vi "Begin.vi"() -> (0 "Error Out":errorcluster)   [LabVIEW 2014]
doc: "Called before other user functions, this VI is expected to open initial I/O refnums, load in file data, and do all program initialization. Notice that the <B>error out</B> terminal is simply used for data flow. Wiring it to other structures or subVIs ensures that this VI runs first."
uses:
  <vilib>/Rock Robotics/WPI/Joystick/WPI_JoystickDeviceEnum.ctl
  <vilib>/Rock Robotics/SystemInterfaces/DIO/FPGA_DIOChannel.ctl
  <vilib>/Rock Robotics/WPI/Solenoid/WPI_SolenoidChannel.ctl
  <vilib>/Rock Robotics/SystemInterfaces/Typedef/FPGA_TypedefDigitalModule.ctl
  <vilib>/Rock Robotics/WPI/Encoder/WPI_EncoderType.ctl
  <vilib>/Rock Robotics/SystemInterfaces/DIO/FPGA_DIOPWMChannel.ctl
  <vilib>/Rock Robotics/SystemInterfaces/AI/FPGA_AIGyroChannel.ctl
  <vilib>/Rock Robotics/SystemInterfaces/Typedef/FPGA_TypedefAnalogModuleForGyro.ctl
  <vilib>/Rock Robotics/SystemInterfaces/Typedef/FPGA_TypedefAnalogModule.ctl
  <vilib>/Rock Robotics/SystemInterfaces/AI/FPGA_AIChannel.ctl
  <vilib>/Rock Robotics/WPI/Solenoid/WPI_SolenoidValue.ctl
  <vilib>/Rock Robotics/WPI/CAN/TalonSRX/WPI_CANTalonSRX_APIControlMode.ctl
  <vilib>/Rock Robotics/WPI/Compressor/WPI_CompressorGetSetRefNum.vi
  <vilib>/Rock Robotics/WPI/Solenoid/WPI_SolenoidOpenDouble.vi
  <vilib>/Rock Robotics/WPI/Counter/WPI_CounterDigitalInputToDigitalSource.vi
  <vilib>/Rock Robotics/WPI/MotorControl/WPI_MotorControlOpen Talon.vi
  <vilib>/Rock Robotics/WPI/MotorControl/WPI_MotorControlOpenCANTalonSRX.vi
  <vilib>/Rock Robotics/WPI/RobotDrive/WPI_RobotDriveOpen4MotorWithExistingMotors.vi
  <vilib>/Rock Robotics/WPI/Solenoid/WPI_SolenoidSetEnum.vi
  <vilib>/Rock Robotics/WPI/RobotDrive/WPI_RobotDriveOpen4MotorWithCANTalonSRX.vi
  <vilib>/Rock Robotics/WPI/CAN/TalonSRX/WPI_CANTalonSRX_BrakeOverride.ctl
panel:
  # "Begin"
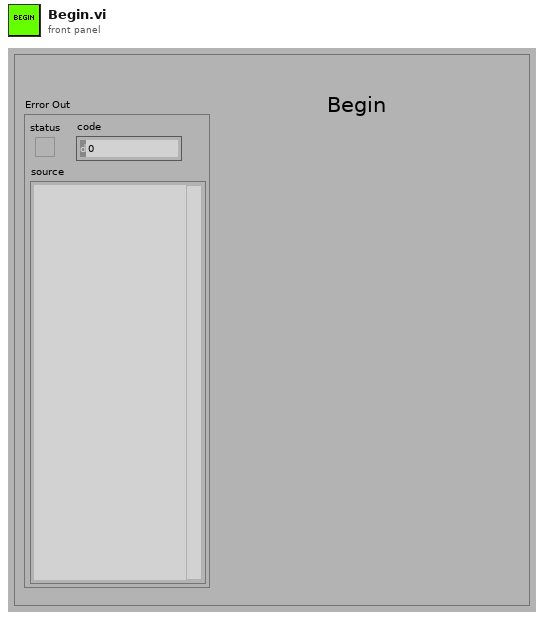
[diagram p1: front panel]
types:
  T1 = typedef "WPI_CANTalonSRX_APIControlMode.ctl" = enum8{"Percent VBus", "Speed", "Position", "Slave", "Unchanged / Invalid"}
  T2 = typedef "WPI_SolenoidValue.ctl" = enum16{"Off", "On", "Forward", "Reverse"}
  T3 = typedef "FPGA_AIChannel.ctl" = enum8{"AI 0", "AI 1", "AI 2", "AI 3", "AI MXP 0", "AI MXP 1", "AI MXP 2", "AI MXP 3", "Invalid"}
  T4 = typedef "FPGA_TypedefAnalogModule.ctl" = enum16{"Controller 1"}
  T5 = typedef "FPGA_TypedefAnalogModuleForGyro.ctl" = enum16{"Controller 1"}
  T6 = typedef "FPGA_AIGyroChannel.ctl" = enum8{"AI 0", "AI 1", "Invalid"}
  T7 = typedef "FPGA_DIOPWMChannel.ctl" = enum8{"PWM 0", "PWM 1", "PWM 2", "PWM 3", "PWM 4", "PWM 5", "PWM 6", "PWM 7", "PWM 8", "PWM 9", "PWM MXP 0", "PWM MXP 1", "PWM MXP 2", "PWM MXP 3", "PWM MXP 4", "PWM MXP 5", "PWM MXP 6", "PWM MXP 7", "PWM MXP 8", "PWM MXP 9", "Invalid"}
  T8 = typedef "WPI_EncoderType.ctl" = enum16{"1x", "2x", "4x"}
  T9 = typedef "FPGA_TypedefDigitalModule.ctl" = enum16{"Controller 1"}
  T10 = typedef "WPI_SolenoidChannel.ctl" = enum8{"Solenoid 0", "Solenoid 1", "Solenoid 2", "Solenoid 3", "Solenoid 4", "Solenoid 5", "Solenoid 6", "Solenoid 7", "Invalid"}
  T11 = typedef "FPGA_DIOChannel.ctl" = enum8{"DIO 0", "DIO 1", "DIO 2", "DIO 3", "DIO 4", "DIO 5", "DIO 6", "DIO 7", "DIO 8", "DIO 9", "DIO MXP 0", "DIO MXP 1", "DIO MXP 2", "DIO MXP 3", "DIO MXP 4", "DIO MXP 5", "DIO MXP 6", "DIO MXP 7", "DIO MXP 8", "DIO MXP 9", "DIO MXP 10", "DIO MXP 11", "DIO MXP 12", "DIO MXP 13", "DIO MXP 14", "DIO MXP 15", "Invalid"}
  T12 = typedef "WPI_JoystickDeviceEnum.ctl" = enum16{"USB 0", "USB 1", "USB 2", "USB 3", "USB 4", "USB 5"}
  T13 = typedef "WPI_RobotDriveDevRef.ctl" = cluster{"DevStatus":errorcluster, "Motors[]":T14[], "Square Inputs":bool, "Max Output":dbl}
  T14 = typedef "WPI_MotorControlDeviceRef.ctl" = cluster{"DeviceStatus":errorcluster, "Type":T15, "PWM":cluster{"Controller":T9, "PWM Channel":T7, "DeadBand":T16}, "CAN":cluster{"Device Number":u8, "Control Mode":T17, "Semaphore":T18, "Max Vout":dbl, "TalonSRX Control Mode":T1}, "Invert":bool, "TransformRef":T19, "InvTransformRef":T19}
  T15 = typedef "WPI_MotorControlType.ctl" = enum16{"PWM", "CAN", "CANTalonSRX"}
  T16 = typedef "WPI_PWMDeadband.ctl" = cluster{"Name":string, "maxPositivePwm":i32, "minPositivePwm":i32, "centerPwm":i32, "maxNegativePwm":i32, "minNegativePwm":i32, "angularRange":u16}
  T17 = typedef "WPI_CANJaguar_ControlMode.ctl" = enum8{"Percent VBus", "Current", "Speed", "Position", "Voltage"}
  T18 = typedef "Semaphore RefNum" = refnum<k1>
  T19 = typedef "WPI_PWMTransform_ConPane.ctl" = refnum<vi>
  T20 = typedef "WPI_CANTalonSRX_BrakeOverride.ctl" = enum8{"No Override", "Override to Coast", "Override to Brake"}
  T21 = typedef "WPI_CompressorDevRef.ctl" = cluster{"DevStatus":errorcluster, "Pneumatics Control Module":u8}
  T22 = typedef "WPI_DigitalInputDevRef.ctl" = cluster{"DevStatus":errorcluster, "DIO Channel":T11, "Controller":T9}
  T23 = typedef "WPI_GyroDevRef.ctl" = cluster{"DevStatus":errorcluster, "Analog Module":T4, "Analog Channel":T3, "Offset":dbl, "Gain (VoltsPerDegree/Second)":dbl}
  T24 = typedef "WPI_AnalogChannelDevRef.ctl" = cluster{"DevStatus":errorcluster, "Controller":T4, "Analog Channel":T3}
  T25 = typedef "WPI_JoystickDevRef.ctl" = cluster{"Device":T12}
  T26 = typedef "WPI_SolenoidDevRef.ctl" = cluster{"DevStatus":errorcluster, "Pneumatics Control Module":u8, "Forward Solenoid Channel":T10, "Reverse Solenoid Channel":T10}
  T27 = typedef "FPGA_CounterEncoderSourceConvertionLVSourceType.ctl" = cluster{"DevStatus":errorcluster, "AnalogTriggerMode?":bool, "DigitalMode":cluster{"Controller":T9, "DIO Channel":T28}, "AnalogTriggerMode":cluster{"AnalogTriggerIndex":T29, "OutputType":T30}}
  T28 = typedef "FPGA_DIODigitalSourceChannel.ctl" = enum8{"DIO 0", "DIO 1", "DIO 2", "DIO 3", "DIO 4", "DIO 5", "DIO 6", "DIO 7", "DIO 8", "DIO 9", "DIO MXP 0", "DIO MXP 1", "DIO MXP 2", "DIO MXP 3", "DIO MXP 4", "DIO MXP 5", "DIO MXP 6", "DIO MXP 7", "DIO MXP 8", "DIO MXP 9", "DIO MXP 10", "DIO MXP 11", "DIO MXP 12", "DIO MXP 13", "DIO MXP 14", "DIO MXP 15", "Disabled"}
  T29 = typedef "FPGA_AnalogTriggerIndex.ctl" = enum8{"Trig 0", "Trig 1", "Trig 2", "Trig 3", "Trig 4", "Trig 5", "Trig 6", "Trig 7", "Invalid"}
  T30 = typedef "FPGA_AnalogTriggerOutType.ctl" = enum16{"InWindow", "TriggerState", "Rising", "Falling"}
  T31 = typedef "WPI_EncoderDevRef.ctl" = cluster{"DevStatus":errorcluster, "EncoderIndex":T32, "CounterIndex":T33, "DistancePerCount":dbl, "Decoding Type":T8}
  T32 = typedef "FPGA_EncoderIdx.ctl" = enum8{"Enc 0", "Enc 1", "Enc 2", "Enc 3", "Enc 4", "Enc 5", "Enc 6", "Enc 7", "Invalid"}
  T33 = typedef "FPGA_CounterCtrSystemIndex.ctl" = enum8{"Ctr 0", "Ctr 1", "Ctr 2", "Ctr 3", "Ctr 4", "Ctr 5", "Ctr 6", "Ctr 7", "Invalid"}
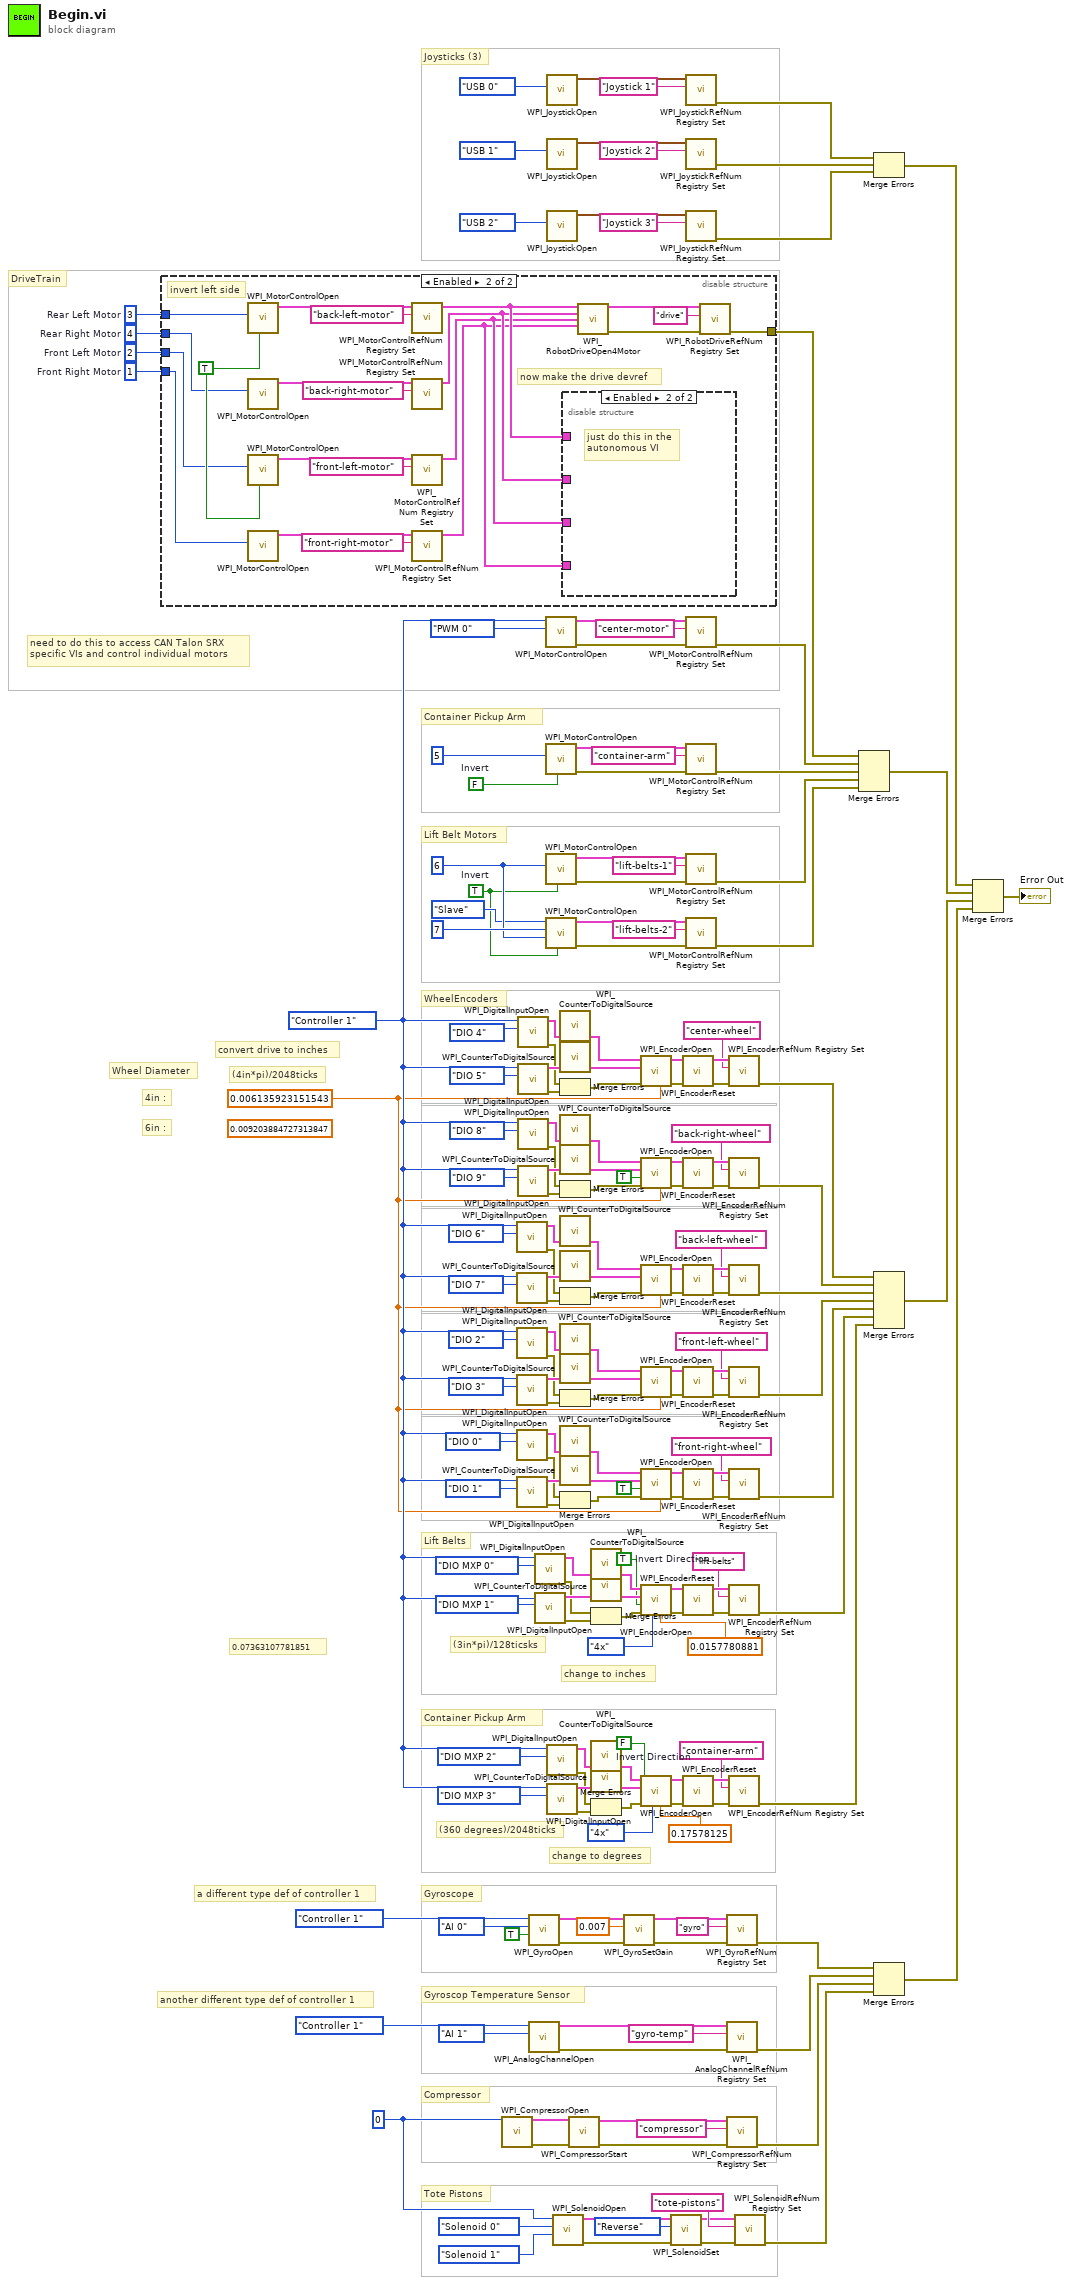
[diagram p0: block diagram]
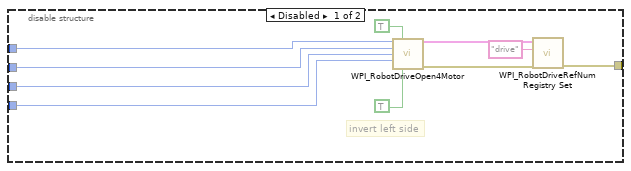
[diagram p2: hidden frame]
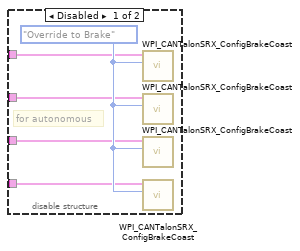
[diagram p3: hidden frame]
diagram:
  w5 = TRUE  # Invert
  w7 = FALSE  # Invert
  w8 = TRUE  # Invert Direction
  w9 = FALSE  # Invert Direction
  (unwired) 0.009203884727313847 ("DistancePerCount")
  w19 = 0.006135923151543 ("DistancePerCount")
  w3 = u8 1  # Front Right Motor
  w4 = u8 2  # Front Left Motor
  w2 = u8 4  # Rear Right Motor
  w1 = u8 3  # Rear Left Motor
  w17 = u8 6 ("Device Number")
  w39 = FPGA_TypedefDigitalModule."Controller 1" ("Controller")
  w18 = u8 0 ("Pneumatics Control Module (0)")
  # "0.07363107781851"
  # "(360 degrees)/2048ticks"
  # "(3in*pi)/128ticsks"
  # "Wheel Diameter"
  # "6in :"
  # "4in :"
  # "convert drive to inches"
  # "(4in*pi)/2048ticks"
  # "need to do this to access CAN Talon SRX\nspecific VIs and control individual motors"
  # "another different type def of controller 1"
  # "Gyroscop Temperature Sensor"
  # "a different type def of controller 1"
  # "Gyroscope"
  # "Lift Belt Motors"
  # "Container Pickup Arm"
  # "DriveTrain"
  # "change to inches"
  # "change to degrees"
  # "Compressor"
  # "Tote Pistons"
  # "Container Pickup Arm"
  # "Lift Belts"
  # "WheelEncoders"
  # "Joysticks (3)"
  n1 = disable-structure shown="Enabled" {
    disable-tunnel: [w199 w211] -> w45
    disable-tunnel: w1 -> [w196 w210]
    disable-tunnel: w2 -> [w195 w209]
    disable-tunnel: w4 -> [w194 w208]
    disable-tunnel: w3 -> [w193 w207]
    frame Disabled {
      # "invert left side"
      n2 = call-poly <vilib>:"WPI_RobotDriveOpen4Motor.vi"("Rear Left Motor"=w196, "Rear Left Motor Inverted"=TRUE, "Rear Right Motor"=w195, "Front Left Motor"=w194, "Front Right Motor"=w193, "Front Left Motor Inverted"=TRUE) -> ("RobotDriveDevRef"=w201:T13, "error out"=w202:errorcluster)  [unwired: 8 in]
      n3 = call <vilib>:"WPI_RobotDriveRefNum Registry Set.vi"("error in (no error)"=w202, "refnum name"="drive", "RobotDriveDevRef"=w201) -> ("error out"=w199:errorcluster)  [unwired: 7 in, 1 out]
    }
    frame Enabled {
      w223 = TRUE ("Invert")
      # "now make the drive devref"
      # "invert left side"
      n4 = call-poly <vilib>:"WPI_MotorControlOpen.vi"("Invert"=w223, "Device Number"=w210) -> ("MotorControlDeviceRef"=w221:T14)  [unwired: 8 in, 1 out]
      n5 = call-poly <vilib>:"WPI_MotorControlOpen.vi"("Device Number"=w209) -> ("MotorControlDeviceRef"=w222:T14)  [unwired: 9 in, 1 out]
      n6 = call-poly <vilib>:"WPI_MotorControlOpen.vi"("Invert"=w223, "Device Number"=w208) -> ("MotorControlDeviceRef"=w217:T14)  [unwired: 8 in, 1 out]
      n7 = call-poly <vilib>:"WPI_MotorControlOpen.vi"("Device Number"=w207) -> ("MotorControlDeviceRef"=w216:T14)  [unwired: 9 in, 1 out]
      n8 = call <vilib>:"WPI_MotorControlRefNum Registry Set.vi"("refnum name"="back-left-motor", "MotorControlDevRef"=w221) -> ("MotorControlDevRef"=w206:T14)  [unwired: 8 in, 1 out]
      n9 = call <vilib>:"WPI_MotorControlRefNum Registry Set.vi"("refnum name"="back-right-motor", "MotorControlDevRef"=w222) -> ("MotorControlDevRef"=w205:T14)  [unwired: 8 in, 1 out]
      n10 = call <vilib>:"WPI_MotorControlRefNum Registry Set.vi"("refnum name"="front-left-motor", "MotorControlDevRef"=w217) -> ("MotorControlDevRef"=w204:T14)  [unwired: 8 in, 1 out]
      n11 = call <vilib>:"WPI_MotorControlRefNum Registry Set.vi"("refnum name"="front-right-motor", "MotorControlDevRef"=w216) -> ("MotorControlDevRef"=w203:T14)  [unwired: 8 in, 1 out]
      n12 = disable-structure shown="Enabled" {
        disable-tunnel: w206 -> [w227 _]
        disable-tunnel: w205 -> [w226 _]
        disable-tunnel: w204 -> [w225 _]
        disable-tunnel: w203 -> [w224 _]
        frame Disabled {
          w228 = WPI_CANTalonSRX_BrakeOverride."Override to Brake" ("Brake / Coast Mode")
          # "for autonomous"
          n13 = call <vilib>:"WPI_CANTalonSRX_ConfigBrakeCoast.vi"("Brake / Coast Mode"=w228, "CAN Talon SRX Ref"=w227) -> ()  [unwired: 8 in, 2 out]
          n14 = call <vilib>:"WPI_CANTalonSRX_ConfigBrakeCoast.vi"("Brake / Coast Mode"=w228, "CAN Talon SRX Ref"=w226) -> ()  [unwired: 8 in, 2 out]
          n15 = call <vilib>:"WPI_CANTalonSRX_ConfigBrakeCoast.vi"("Brake / Coast Mode"=w228, "CAN Talon SRX Ref"=w225) -> ()  [unwired: 8 in, 2 out]
          n16 = call <vilib>:"WPI_CANTalonSRX_ConfigBrakeCoast.vi"("Brake / Coast Mode"=w228, "CAN Talon SRX Ref"=w224) -> ()  [unwired: 8 in, 2 out]
        }
        frame Enabled {
          # "just do this in the\nautonomous VI"
        }
      }
      n17 = call-poly <vilib>:"WPI_RobotDriveOpen4Motor.vi"("Rear Left Motor Dev Ref"=w206, "Rear Right Motor Dev Ref"=w205, "Front Left Motor Dev Ref"=w204, "Front Right Motor Dev Ref"=w203) -> ("RobotDriveDevRef"=w213:T13, "error out"=w214:errorcluster)  [unwired: 10 in]
      n18 = call <vilib>:"WPI_RobotDriveRefNum Registry Set.vi"("error in (no error)"=w214, "refnum name"="drive", "RobotDriveDevRef"=w213) -> ("error out"=w211:errorcluster)  [unwired: 7 in, 1 out]
    }
  }
  n19 = call <vilib>:"WPI_CompressorOpen.vi"("Pneumatics Control Module (0)"=w18) -> ("CompressorDevRef"=w90:T21, "error out"=w89:errorcluster)  [unwired: 13 in]
  n20 = call <vilib>:"WPI_DigitalInputOpen.vi"("DIO Channel"=FPGA_DIOChannel."DIO 6" ("A Channel"), "Controller"=w39) -> ("error out"=w68:errorcluster, "DigitalInputDevRef"=w157:T22)  [unwired: 1 in, 7 out]
  n21 = call <vilib>:"WPI_DigitalInputOpen.vi"("DIO Channel"=FPGA_DIOChannel."DIO 7" ("B Channel"), "Controller"=w39) -> ("error out"=w69:errorcluster, "DigitalInputDevRef"=w158:T22)  [unwired: 1 in, 7 out]
  n22 = call <vilib>:"WPI_DigitalInputOpen.vi"("DIO Channel"=FPGA_DIOChannel."DIO 2" ("A Channel"), "Controller"=w39) -> ("error out"=w71:errorcluster, "DigitalInputDevRef"=w146:T22)  [unwired: 1 in, 7 out]
  n23 = call <vilib>:"WPI_DigitalInputOpen.vi"("DIO Channel"=FPGA_DIOChannel."DIO 3" ("B Channel"), "Controller"=w39) -> ("error out"=w72:errorcluster, "DigitalInputDevRef"=w145:T22)  [unwired: 1 in, 7 out]
  n24 = call <vilib>:"WPI_DigitalInputOpen.vi"("DIO Channel"=FPGA_DIOChannel."DIO 0" ("A Channel"), "Controller"=w39) -> ("error out"=w74:errorcluster, "DigitalInputDevRef"=w137:T22)  [unwired: 1 in, 7 out]
  n25 = call <vilib>:"WPI_DigitalInputOpen.vi"("DIO Channel"=FPGA_DIOChannel."DIO 1" ("B Channel"), "Controller"=w39) -> ("error out"=w75:errorcluster, "DigitalInputDevRef"=w138:T22)  [unwired: 1 in, 7 out]
  n26 = call <vilib>:"WPI_DigitalInputOpen.vi"("DIO Channel"=FPGA_DIOChannel."DIO 4" ("A Channel"), "Controller"=w39) -> ("error out"=w61:errorcluster, "DigitalInputDevRef"=w179:T22)  [unwired: 1 in, 7 out]
  n27 = call <vilib>:"WPI_DigitalInputOpen.vi"("DIO Channel"=FPGA_DIOChannel."DIO 5" ("B Channel"), "Controller"=w39) -> ("error out"=w63:errorcluster, "DigitalInputDevRef"=w180:T22)  [unwired: 1 in, 7 out]
  n28 = call <vilib>:"WPI_DigitalInputOpen.vi"("DIO Channel"=FPGA_DIOChannel."DIO 8" ("A Channel"), "Controller"=w39) -> ("error out"=w64:errorcluster, "DigitalInputDevRef"=w166:T22)  [unwired: 1 in, 7 out]
  n29 = call <vilib>:"WPI_DigitalInputOpen.vi"("DIO Channel"=FPGA_DIOChannel."DIO 9" ("B Channel"), "Controller"=w39) -> ("error out"=w66:errorcluster, "DigitalInputDevRef"=w165:T22)  [unwired: 1 in, 7 out]
  n30 = call <vilib>:"WPI_GyroOpen.vi"("Calibrate On Open"=TRUE, "Analog Channel"=FPGA_AIGyroChannel."AI 0", "Controller"=FPGA_TypedefAnalogModuleForGyro."Controller 1") -> ("error out"=w35:errorcluster, "GyroDevRef"=w36:T23)  [unwired: 6 in, 1 out]
  n31 = call <vilib>:"WPI_AnalogChannelOpen.vi"("Analog Channel"=FPGA_AIChannel."AI 1", "Controller"=FPGA_TypedefAnalogModule."Controller 1") -> ("error out"=w24:errorcluster, "AIDeviceRef"=w25:T24)  [unwired: 8 in]
  n32 = call <vilib>:"WPI_DigitalInputOpen.vi"("DIO Channel"=FPGA_DIOChannel."DIO MXP 0" ("A Channel"), "Controller"=w39) -> ("error out"=w82:errorcluster, "DigitalInputDevRef"=w126:T22)  [unwired: 1 in, 7 out]
  n33 = call <vilib>:"WPI_DigitalInputOpen.vi"("DIO Channel"=FPGA_DIOChannel."DIO MXP 1" ("B Channel"), "Controller"=w39) -> ("error out"=w81:errorcluster, "DigitalInputDevRef"=w125:T22)  [unwired: 1 in, 7 out]
  n34 = call-poly <vilib>:"WPI_MotorControlOpen.vi"("PWM Channel"=FPGA_DIOPWMChannel."PWM 0", "Controller"=w39) -> ("error out"=w60:errorcluster, "MotorControlDeviceRef"=w59:T14)  [unwired: 8 in]
  n35 = call-poly <vilib>:"WPI_MotorControlOpen.vi"("Invert"=w7, "Device Number"=u8 5) -> ("error out"=w56:errorcluster, "MotorControlDeviceRef"=w57:T14)  [unwired: 8 in]
  n36 = call-poly <vilib>:"WPI_MotorControlOpen.vi"("Invert"=w5, "Device Number"=w17) -> ("error out"=w53:errorcluster, "MotorControlDeviceRef"=w54:T14)  [unwired: 8 in]
  n37 = call-poly <vilib>:"WPI_MotorControlOpen.vi"("Invert"=w5, "Master Device Number"=w17, "Device Number"=u8 7, "Control Mode"=WPI_CANTalonSRX_APIControlMode."Slave") -> ("error out"=w49:errorcluster, "MotorControlDeviceRef"=w48:T14)  [unwired: 6 in]
  n38 = call <vilib>:"WPI_JoystickOpen.vi"("JoystickDevice"=WPI_JoystickDeviceEnum."USB 0") -> ("JoystickDevRef"=w185:T25)  [unwired: 10 in]
  n39 = call <vilib>:"WPI_JoystickOpen.vi"("JoystickDevice"=WPI_JoystickDeviceEnum."USB 1") -> ("JoystickDevRef"=w188:T25)  [unwired: 10 in]
  n40 = call <vilib>:"WPI_JoystickOpen.vi"("JoystickDevice"=WPI_JoystickDeviceEnum."USB 2") -> ("JoystickDevRef"=w191:T25)  [unwired: 10 in]
  n41 = call <vilib>:"WPI_DigitalInputOpen.vi"("DIO Channel"=FPGA_DIOChannel."DIO MXP 2" ("A Channel"), "Controller"=w39) -> ("error out"=w86:errorcluster, "DigitalInputDevRef"=w117:T22)  [unwired: 1 in, 7 out]
  n42 = call <vilib>:"WPI_DigitalInputOpen.vi"("DIO Channel"=FPGA_DIOChannel."DIO MXP 3" ("B Channel"), "Controller"=w39) -> ("error out"=w87:errorcluster, "DigitalInputDevRef"=w118:T22)  [unwired: 1 in, 7 out]
  n43 = call-poly <vilib>:"WPI_SolenoidOpen.vi"("Reverse Solenoid Channel"=WPI_SolenoidChannel."Solenoid 1", "Forward Solenoid Channel"=WPI_SolenoidChannel."Solenoid 0", "Pneumatics Control Module (0)"=w18) -> ("error out"=w14:errorcluster, "SolenoidDevRef"=w13:T26)  [unwired: 7 in]
  n44 = call-poly <vilib>:"WPI_CounterToDigitalSource.vi"("DigitalInputDevRef"=w179) -> ("Digital Source"=w178:T27)  [unwired: 6 out]
  n45 = call-poly <vilib>:"WPI_CounterToDigitalSource.vi"("DigitalInputDevRef"=w180) -> ("Digital Source"=w181:T27)  [unwired: 6 out]
  n46 = Merge Errors(w61, w63) -> (w62:errorcluster)
  n47 = call-poly <vilib>:"WPI_CounterToDigitalSource.vi"("DigitalInputDevRef"=w166) -> ("Digital Source"=w167:T27)  [unwired: 6 out]
  n48 = call-poly <vilib>:"WPI_CounterToDigitalSource.vi"("DigitalInputDevRef"=w165) -> ("Digital Source"=w164:T27)  [unwired: 6 out]
  n49 = Merge Errors(w64, w66) -> (w65:errorcluster)
  n50 = call-poly <vilib>:"WPI_CounterToDigitalSource.vi"("DigitalInputDevRef"=w157) -> ("Digital Source"=w156:T27)  [unwired: 6 out]
  n51 = call-poly <vilib>:"WPI_CounterToDigitalSource.vi"("DigitalInputDevRef"=w158) -> ("Digital Source"=w159:T27)  [unwired: 6 out]
  n52 = Merge Errors(w68, w69) -> (w67:errorcluster)
  n53 = call-poly <vilib>:"WPI_CounterToDigitalSource.vi"("DigitalInputDevRef"=w146) -> ("Digital Source"=w147:T27)  [unwired: 6 out]
  n54 = call-poly <vilib>:"WPI_CounterToDigitalSource.vi"("DigitalInputDevRef"=w145) -> ("Digital Source"=w144:T27)  [unwired: 6 out]
  n55 = Merge Errors(w71, w72) -> (w70:errorcluster)
  n56 = call-poly <vilib>:"WPI_CounterToDigitalSource.vi"("DigitalInputDevRef"=w137) -> ("Digital Source"=w136:T27)  [unwired: 6 out]
  n57 = call-poly <vilib>:"WPI_CounterToDigitalSource.vi"("DigitalInputDevRef"=w138) -> ("Digital Source"=w139:T27)  [unwired: 6 out]
  n58 = Merge Errors(w74, w75) -> (w73:errorcluster)
  n59 = call <vilib>:"WPI_CompressorStart.vi"("error in (no error)"=w89, "CompressorDevRef"=w90) -> ("error out"=w172:errorcluster, "CompressorDevRef"=w173:T21)  [unwired: 8 in]
  n60 = call-poly <vilib>:"WPI_CounterToDigitalSource.vi"("DigitalInputDevRef"=w126) -> ("Digital Source"=w127:T27)  [unwired: 6 out]
  n61 = call-poly <vilib>:"WPI_CounterToDigitalSource.vi"("DigitalInputDevRef"=w125) -> ("Digital Source"=w124:T27)  [unwired: 6 out]
  n62 = Merge Errors(w82, w81) -> (w83:errorcluster)
  n63 = call-poly <vilib>:"WPI_CounterToDigitalSource.vi"("DigitalInputDevRef"=w117) -> ("Digital Source"=w116:T27)  [unwired: 6 out]
  n64 = call-poly <vilib>:"WPI_CounterToDigitalSource.vi"("DigitalInputDevRef"=w118) -> ("Digital Source"=w119:T27)  [unwired: 6 out]
  n65 = Merge Errors(w86, w87) -> (w88:errorcluster)
  n66 = call <vilib>:"WPI_GyroSetGain.vi"("error in (no error)"=w35, "Gain (VoltsPerDegree/Second)"=0.007, "GyroDevRef"=w36) -> ("error out"=w34:errorcluster, "GyroDevRef"=w33:T23)  [unwired: 7 out]
  n67 = call <vilib>:"WPI_EncoderOpen.vi"("DistancePerCount"=w19, "error in (no error)"=w62, "BSource"=w181, "ASource"=w178) -> ("error out"=w176:errorcluster, "EncoderDevRef"=w177:T31)  [unwired: 4 in, 2 out]
  n68 = call <vilib>:"WPI_EncoderOpen.vi"("DistancePerCount"=w19, "error in (no error)"=w65, "Invert Direction (False)"=TRUE, "BSource"=w164, "ASource"=w167) -> ("error out"=w169:errorcluster, "EncoderDevRef"=w168:T31)  [unwired: 3 in, 2 out]
  n69 = call <vilib>:"WPI_EncoderOpen.vi"("DistancePerCount"=w19, "error in (no error)"=w67, "BSource"=w159, "ASource"=w156) -> ("error out"=w154:errorcluster, "EncoderDevRef"=w155:T31)  [unwired: 4 in, 2 out]
  n70 = call <vilib>:"WPI_EncoderOpen.vi"("DistancePerCount"=w19, "error in (no error)"=w70, "BSource"=w144, "ASource"=w147) -> ("error out"=w149:errorcluster, "EncoderDevRef"=w148:T31)  [unwired: 4 in, 2 out]
  n71 = call <vilib>:"WPI_EncoderOpen.vi"("DistancePerCount"=w19, "error in (no error)"=w73, "Invert Direction (False)"=TRUE, "BSource"=w139, "ASource"=w136) -> ("error out"=w134:errorcluster, "EncoderDevRef"=w135:T31)  [unwired: 3 in, 2 out]
  n72 = call <vilib>:"WPI_EncoderOpen.vi"("DistancePerCount"=0.0157780881, "Decoding Type"=WPI_EncoderType."4x", "error in (no error)"=w83, "Invert Direction (False)"=w8, "BSource"=w124, "ASource"=w127) -> ("error out"=w129:errorcluster, "EncoderDevRef"=w128:T31)  [unwired: 2 in, 2 out]
  n73 = call <vilib>:"WPI_EncoderOpen.vi"("DistancePerCount"=0.17578125, "Decoding Type"=WPI_EncoderType."4x", "error in (no error)"=w88, "Invert Direction (False)"=w9, "BSource"=w119, "ASource"=w116) -> ("error out"=w114:errorcluster, "EncoderDevRef"=w115:T31)  [unwired: 2 in, 2 out]
  n74 = call-poly <vilib>:"WPI_SolenoidSet.vi"("error in (no error)"=w14, "Value"=WPI_SolenoidValue."Reverse", "SolenoidDevRef"=w13) -> ("error out"=w15:errorcluster, "SolenoidDevRef"=w12:T26)  [unwired: 7 in]
  n75 = call <vilib>:"WPI_EncoderReset.vi"("error in (no error)"=w176, "EncoderDevRef"=w177) -> ("error out"=w175:errorcluster, "EncoderDevRef"=w174:T31)  [unwired: 8 in]
  n76 = call <vilib>:"WPI_EncoderReset.vi"("error in (no error)"=w169, "EncoderDevRef"=w168) -> ("error out"=w170:errorcluster, "EncoderDevRef"=w171:T31)  [unwired: 8 in]
  n77 = call <vilib>:"WPI_EncoderReset.vi"("error in (no error)"=w154, "EncoderDevRef"=w155) -> ("error out"=w153:errorcluster, "EncoderDevRef"=w152:T31)  [unwired: 8 in]
  n78 = call <vilib>:"WPI_EncoderReset.vi"("error in (no error)"=w149, "EncoderDevRef"=w148) -> ("error out"=w150:errorcluster, "EncoderDevRef"=w151:T31)  [unwired: 8 in]
  n79 = call <vilib>:"WPI_EncoderReset.vi"("error in (no error)"=w134, "EncoderDevRef"=w135) -> ("error out"=w133:errorcluster, "EncoderDevRef"=w132:T31)  [unwired: 8 in]
  n80 = call <vilib>:"WPI_EncoderReset.vi"("error in (no error)"=w129, "EncoderDevRef"=w128) -> ("error out"=w130:errorcluster, "EncoderDevRef"=w131:T31)  [unwired: 8 in]
  n81 = call <vilib>:"WPI_EncoderReset.vi"("error in (no error)"=w114, "EncoderDevRef"=w115) -> ("error out"=w113:errorcluster, "EncoderDevRef"=w112:T31)  [unwired: 8 in]
  n82 = call <vilib>:"WPI_JoystickRefNum Registry Set.vi"("refnum name"="Joystick 1", "JoystickDevRef"=w185) -> ("error out"=w91:errorcluster)  [unwired: 8 in, 1 out]
  n83 = call <vilib>:"WPI_JoystickRefNum Registry Set.vi"("refnum name"="Joystick 2", "JoystickDevRef"=w188) -> ("error out"=w92:errorcluster)  [unwired: 8 in, 1 out]
  n84 = call <vilib>:"WPI_JoystickRefNum Registry Set.vi"("refnum name"="Joystick 3", "JoystickDevRef"=w191) -> ("error out"=w93:errorcluster)  [unwired: 8 in, 1 out]
  n85 = call <vilib>:"WPI_MotorControlRefNum Registry Set.vi"("error in (no error)"=w60, "refnum name"="center-motor", "MotorControlDevRef"=w59) -> ("error out"=w46:errorcluster)  [unwired: 7 in, 1 out]
  n86 = call <vilib>:"WPI_MotorControlRefNum Registry Set.vi"("error in (no error)"=w56, "refnum name"="container-arm", "MotorControlDevRef"=w57) -> ("error out"=w47:errorcluster)  [unwired: 7 in, 1 out]
  n87 = call <vilib>:"WPI_MotorControlRefNum Registry Set.vi"("error in (no error)"=w53, "refnum name"="lift-belts-1", "MotorControlDevRef"=w54) -> ("error out"=w29:errorcluster)  [unwired: 7 in, 1 out]
  n88 = call <vilib>:"WPI_MotorControlRefNum Registry Set.vi"("error in (no error)"=w49, "refnum name"="lift-belts-2", "MotorControlDevRef"=w48) -> ("error out"=w28:errorcluster)  [unwired: 7 in, 1 out]
  n89 = call <vilib>:"WPI_GyroRefNum Registry Set.vi"("error in (no error)"=w34, "refnum name"="gyro", "GyroDevRef"=w33) -> ("error out"=w30:errorcluster)  [unwired: 7 in, 1 out]
  n90 = call <vilib>:"WPI_AnalogChannelRefNum Registry Set.vi"("error in (no error)"=w24, "refnum name"="gyro-temp", "AIDeviceRef"=w25) -> ("error out"=w20:errorcluster)  [unwired: 7 in, 1 out]
  n91 = call <vilib>:"WPI_CompressorRefNum Registry Set.vi"("error in (no error)"=w172, "refnum name"="compressor", "CompressorDevRef"=w173) -> ("error out"=w21:errorcluster)  [unwired: 7 in, 1 out]
  n92 = call <vilib>:"WPI_EncoderRefNum Registry Set.vi"("error in (no error)"=w175, "refnum name"="center-wheel", "EncoderDevRef"=w174) -> ("error out"=w95:errorcluster)  [unwired: 7 in, 1 out]
  n93 = call <vilib>:"WPI_EncoderRefNum Registry Set.vi"("error in (no error)"=w170, "refnum name"="back-right-wheel", "EncoderDevRef"=w171) -> ("error out"=w96:errorcluster)  [unwired: 7 in, 1 out]
  n94 = call <vilib>:"WPI_EncoderRefNum Registry Set.vi"("error in (no error)"=w153, "refnum name"="back-left-wheel", "EncoderDevRef"=w152) -> ("error out"=w97:errorcluster)  [unwired: 7 in, 1 out]
  n95 = call <vilib>:"WPI_EncoderRefNum Registry Set.vi"("error in (no error)"=w150, "refnum name"="front-left-wheel", "EncoderDevRef"=w151) -> ("error out"=w98:errorcluster)  [unwired: 7 in, 1 out]
  n96 = call <vilib>:"WPI_EncoderRefNum Registry Set.vi"("error in (no error)"=w133, "refnum name"="front-right-wheel", "EncoderDevRef"=w132) -> ("error out"=w99:errorcluster)  [unwired: 7 in, 1 out]
  n97 = call <vilib>:"WPI_EncoderRefNum Registry Set.vi"("error in (no error)"=w130, "refnum name"="lift-belts", "EncoderDevRef"=w131) -> ("error out"=w78:errorcluster)  [unwired: 7 in, 1 out]
  n98 = call <vilib>:"WPI_EncoderRefNum Registry Set.vi"("error in (no error)"=w113, "refnum name"="container-arm", "EncoderDevRef"=w112) -> ("error out"=w76:errorcluster)  [unwired: 7 in, 1 out]
  n99 = call <vilib>:"WPI_SolenoidRefNum Registry Set.vi"("error in (no error)"=w15, "refnum name"="tote-pistons", "SolenoidDevRef"=w12) -> ("error out"=w22:errorcluster)  [unwired: 7 in, 1 out]
  n100 = Merge Errors(w45, w46, w47, w29, w28) -> (w43:errorcluster)
  n101 = Merge Errors(w91, w92, w93) -> (w44:errorcluster)
  n102 = Merge Errors(w95, w96, w97, w98, w99, w78, w76) -> (w94:errorcluster)
  n103 = Merge Errors(w30, w20, w21, w22) -> (w77:errorcluster)
  n104 = Merge Errors(w44, w43, w94, w77) -> (→"Error Out":errorcluster)
